vi "Launch Rooms Manager.vi"(0 "Hotel Management Tool Model in":refnum<class "Hotel Management Tool Model.lvclass">, 11 "error in (no error)":errorcluster) -> (4 "Hotel Management Tool Model out":refnum<class "Hotel Management Tool Model.lvclass">, 15 "error out":errorcluster)   [LabVIEW 2023, in "Hotel Management Tool Model.lvlib" / "Hotel Management Tool Model.lvclass"]
uses:
  Hotel Management Tool Model.lvclass
  Rooms Manager Model/Rooms Manager Model/Rooms Manager Model.lvclass
  Hotel Management Tool Model.lvclass/Hotel Management Tool Model.ctl
  <vilib>/ActorFramework/Message Enqueuer/Message Enqueuer.lvclass/Message Enqueuer.ctl
  <vilib>/ActorFramework/Message Enqueuer/Enqueue.vi
  Central Data Manager/Central Data Manager Messages/Refresh Rooms Status Msg/Refresh Rooms Status Msg.lvclass
  <vilib>/ActorFramework/Message Priority Queue/Priority Enqueue.vi
  <vilib>/ActorFramework/Actor/Actor.lvclass
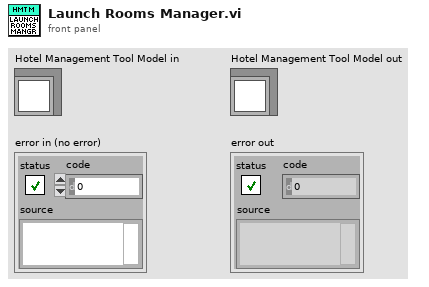
[diagram p1: front panel]
types:
  T1 = map{string, refnum<class "Message Enqueuer.lvclass">}
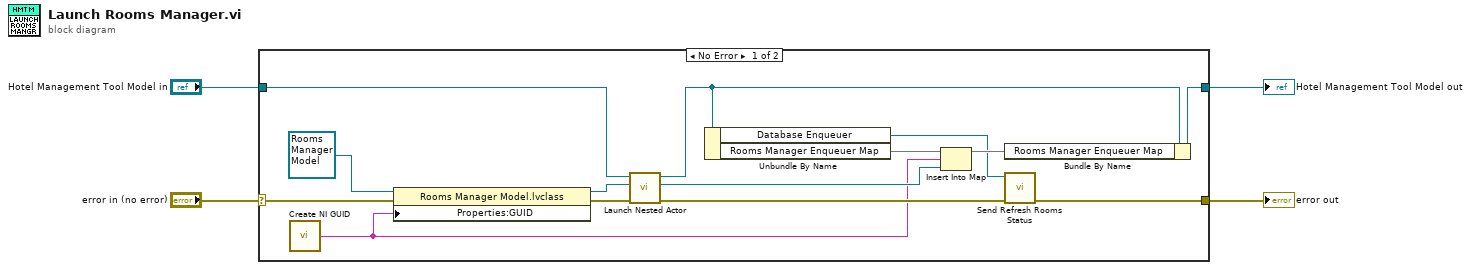
[diagram p0: block diagram]
diagram:
  n1 = case shown="No Error" "error in (no error)" {
    selector: "error in (no error)" -> [w18 w20]
    tunnel: [w12 w20] -> w3
    tunnel: [w15 w19] -> w1
    tunnel: "Hotel Management Tool Model in" -> [w17 w19]
    frame No Error {
      n2 = call <vilib>:"Create NI GUID.vi"() -> ("NI GUID"=w6:string)
      n3 = property class="Rooms Manager Model.lvclass"(reference=refnum<class "Rooms Manager Model.lvclass"> refnum ("Rooms Manager Model.lvlib:Rooms Manager Model.lvclass"), error in=w18, "Properties:GUID"=w6) -> (reference out=w9:refnum<class "Rooms Manager Model.lvclass">, error out=w11:errorcluster)
      n4 = call <vilib>:"Launch Nested Actor.vi"("error in (no error)"=w11, "Nested Actor"=w9, "Caller Actor in"=w17) -> ("error out"=w13:errorcluster, "Nested Actor's Enqueuer"=w14:refnum<class "Message Enqueuer.lvclass">, "Caller Actor out"=w16:refnum<class "Hotel Management Tool Model.lvclass">)  [unwired: 6 in]
      n5 = Unbundle By Name(w16) -> ("Database Enqueuer"=w5:refnum<class "Message Enqueuer.lvclass">, "Rooms Manager Enqueuer Map"=w7:T1)
      n6 = Insert Into Map(map in=w7, key=w6, value=w14) -> (map out=w8:T1)  [unwired: 2 out]
      n7 = Bundle By Name(cluster=w16, "Rooms Manager Enqueuer Map"=w8) -> (w15:refnum<class "Hotel Management Tool Model.lvclass">)
      n8 = call "Send Refresh Rooms Status.vi"("error in (no error)"=w13, "Message Enqueuer"=w5) -> ("error out"=w12:errorcluster)  [unwired: 8 in, 1 out]
    }
    frame Error {
    }
  }
  "error out" <- w3
  "Hotel Management Tool Model out" <- w1
